vi "main_remote_FPGA.vi"() -> ()   [LabVIEW 2019]
uses:
  <vilib>/platform/TimedLoop/XDataNode/XDataNode.xnode
  <vilib>/Platform/TimedLoop/XDataNode/nitl_modes.ctl
  <vilib>/Platform/TimedLoop/XDataNode/XDNodeRunTimeDep.lvlib
  <vilib>/Platform/TimedLoop/XDataNode/wakeup.ctl
  <vilib>/Platform/TimedLoop/XDataNode/timing_clust.ctl
  FPGA_subVIs/old/motor/motor single class/Variable PID(Kp) mode enum.ctl
  FPGA_subVIs/old/motor/motor single class/Motor single.lvclass
  FPGA_subVIs/old/motor/motor single class/Variable PID(Kp).ctl
  FPGA_subVIs/old/motor/motor enum(FPGA).ctl
panel:
  out "Waveform Chart 2":dbl(graph)
  out "Waveform Chart":cluster{"setpoint":dbl, "encoder out":i32}(graph)
  out "PID out":dbl[](array[numeric])
  out "encoder":i32[](array[numeric])
  out "setpoint":dbl[](array[numeric])
  in  "stop":bool
  out "error out":errorcluster
  in  "error in (no error)":errorcluster
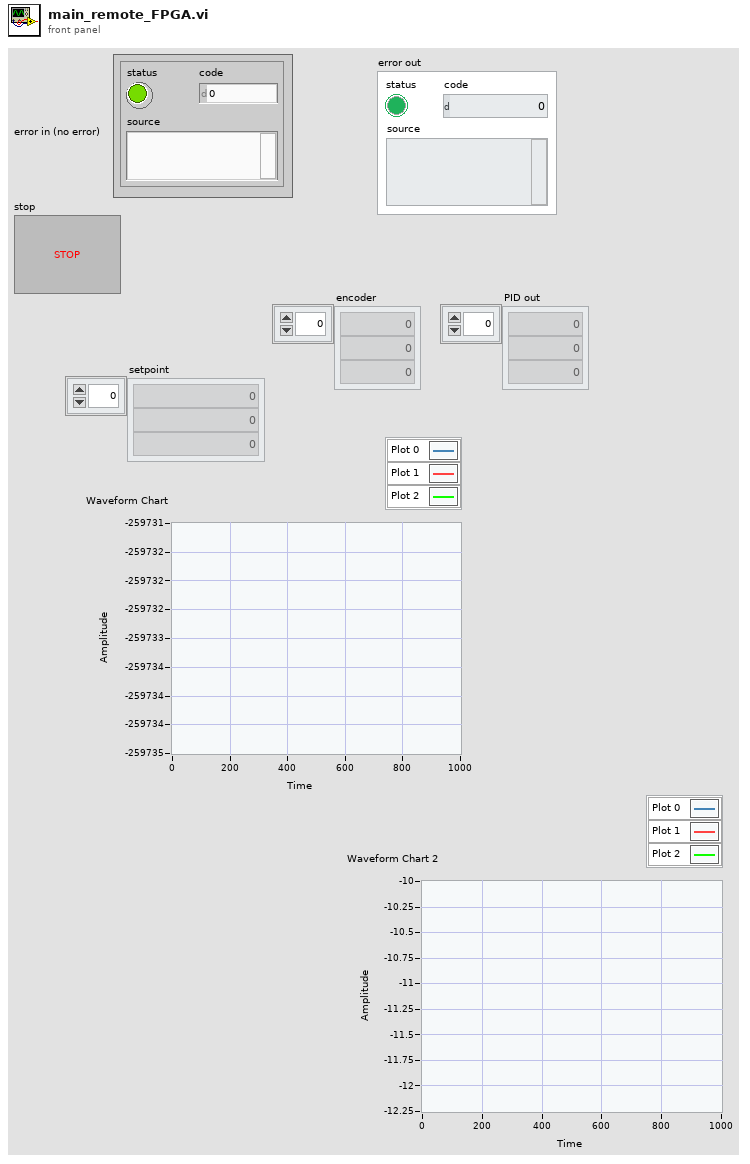
[diagram p1: front panel]
types:
  T1 = typedef "Motor single.lvclass/motor enum(FPGA).ctl" = enum16{"M1", "M2", "M3", "M4"}
  T2 = typedef "Motor single.lvclass/Variable PID(Kp).ctl" = cluster{"Enable variable PID(Kp)":bool, "Variable PID(Kp)range":dbl, "Variable MODE":T3}
  T3 = typedef "Motor single.lvclass/Variable PID(Kp) mode enum.ctl" = enum16{"Log", "Sin&Cos", "Linear", "reverse Log", "const"}
  T4 = typedef "XDNodeRunTimeDep.lvlib/timing_clust.ctl" = cluster{"Expected End [f-1]":u64, "Actual End [f-1]":u64, "Finished Late? [f-1]":bool, "Expected End [i-1]":u64, "Actual End [i-1]":u64, "Finished Late? [i-1]":bool, "Expected Start [i]":u64, "Actual Start [i]":u64, "Expected Start [f]":u64, "Actual Start [f]":u64, "Source Name":string, "Structure Name":string, "Period":i64, "Deadline":i64, "Offset":i64, "Start":i64, "Priority":i32, "Timeout":i32, "Mode":T5, "Wakeup Reason":T6, "Error":errorcluster, "Source Type":string, "Secondary Source Type":string, "Global End Time":u64, "Global Start Time":u64, "Frame Duration":u64, "Iteration Duration":u64, "Assigned CPU":i32, "I/O Scan Engine Mode":u32}
  T5 = typedef "XDNodeRunTimeDep.lvlib/nitl_modes.ctl" = enum32{"No Change", "Process missed periods, maintain original phase", "Discard missed periods, maintain original phase", "Process missed periods, ignore original phase", "Discard missed periods, ignore original phase"}
  T6 = typedef "XDNodeRunTimeDep.lvlib/wakeup.ctl" = enum32{"Normal", "Aborted", "Asynchronous wakeup", "Timing source error", "Timed loop error", "Timeout"}
  T7 = typedef "f710.ctl" = cluster{"Down":bool, "Left":bool, "Up":bool, "Right":bool, "A":bool, "X":bool, "Y":bool, "B":bool, "LB":bool, "RB":bool, "LT":i16, "RT":i16, "L3":bool, "R3":bool, "Ly":i16, "Lx":i16, "Ry":i16, "Rx":i16, "Back":bool, "Start":bool, "center":bool}
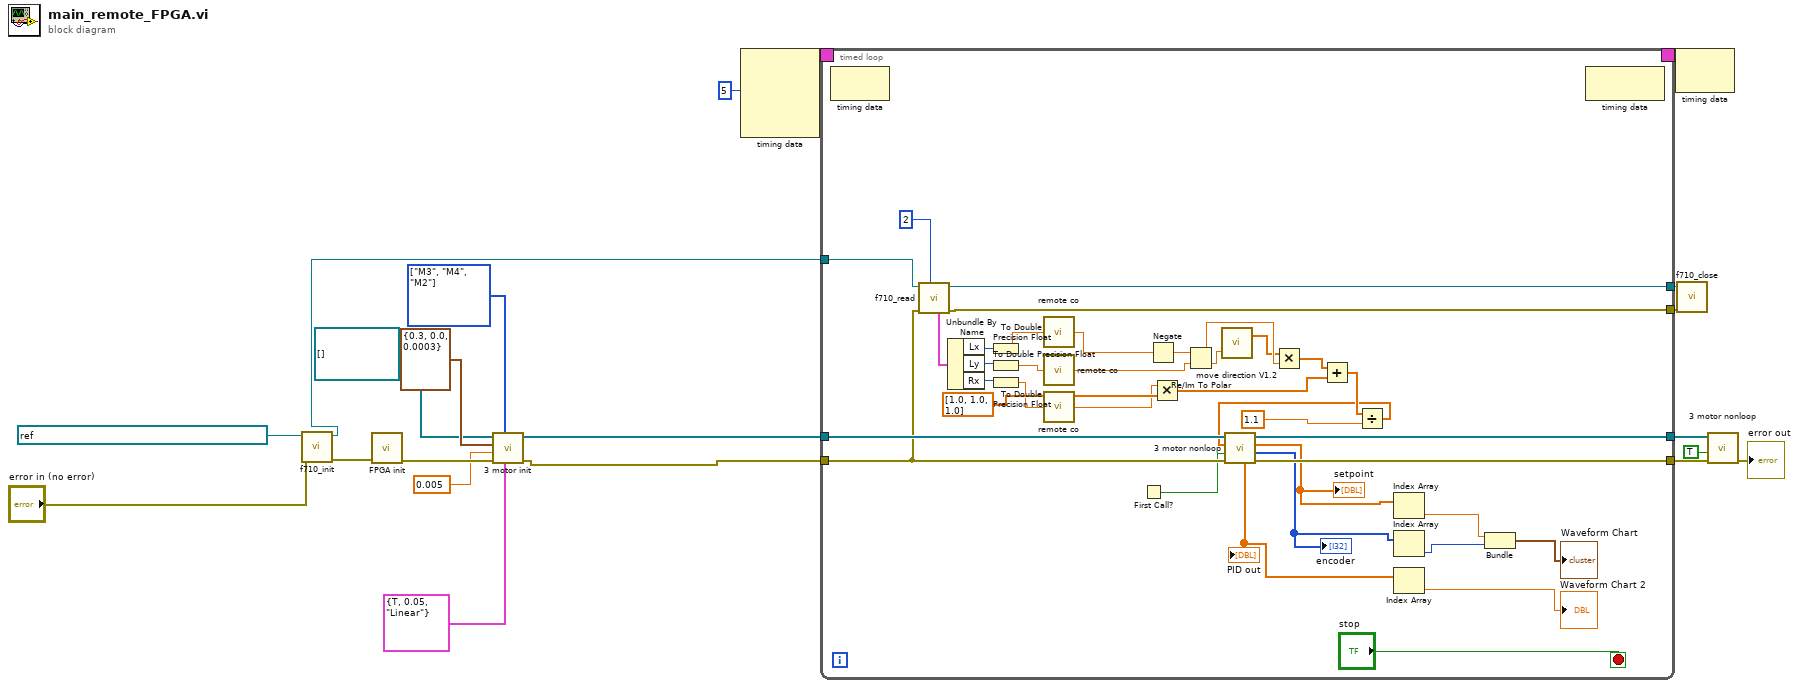
[diagram p0: block diagram]
diagram:
  w12 = T1[] [enum."M3", enum."M4", enum."M2"] items=["M1", "M2", "M3", "M4"] ("Array 2")
  n1 = call <userlib>:"f710_init.vi"("error in (no error)"="error in (no error)", "USB RAW VISA resource name"=refnum<visa-resource-name> "USB0::0x046D::0xC21F::EEAB948F::RAW") -> ("error out"=w5:errorcluster, "VISA Refnum out"=w8:refnum<visa-resource-name>)  [unwired: 8 in]
  n2 = call "FPGA init.vi"("error in"=w5) -> ("error out"=w18:errorcluster)  [unwired: 9 in, 1 out]
  n3 = call "3 motor init.vi"("Variable PID(Kp)"=T2 {"Enable variable PID(Kp)"=TRUE, "Variable PID(Kp)range"=0.05, "Variable MODE"=enum."Linear"}, "Array 2"=w12, "Error In"=w18, "dt(s)"=0.005, "PID"=cluster{"Kp":dbl, "Ki":dbl, "Kd":dbl} {"Kp"=0.3, "Ki"=0.0, "Kd"=0.0003}, "Array"=refnum<class "Motor single.lvclass">[] []) -> ("error out"=w19:errorcluster, "Object array"=w17:refnum<class "Motor single.lvclass">[])  [unwired: 4 in]
  n4 = node-c288(i64 5 ("Period")) -> (w21:T4)  [unwired: 3 in]
  n5 = timed-loop {
    timing: w21 -> [_]
    timing-out: [_] -> w20
    tunnel: w19 -> [w54]
    tunnel: w17 -> [w58]
    tunnel: [w57] -> w11
    tunnel: [w56] -> w10
    tunnel: w8 -> [w55]
    tunnel: [w53] -> w4
    tunnel: [w52] -> w1
    stop <- "stop" stop-if-true
    n6 = node-c288() -> ()  [unwired: 1 in, 1 out]
    n7 = call <userlib>:"f710_read.vi"("Timeout to wait for Interrupt (ms)"=u32 2, "error in (no error)"=w54, "VISA Refnum in"=w55) -> ("error out"=w57:errorcluster, "VISA Refnum out"=w56:refnum<visa-resource-name>, "F710"=w33:T7)  [unwired: 6 in]
    n8 = Unbundle By Name(w33) -> ("Lx"=w51:i16, "Ly"=w50:i16, "Rx"=w49:i16)
    n9 = To Double Precision Float(number=w51) -> (double precision float=w39:dbl)
    n10 = To Double Precision Float(number=w50) -> (double precision float=w37:dbl)
    n11 = To Double Precision Float(number=w49) -> (double precision float=w34:dbl)
    n12 = call "remote co.vi"("input"=w39) -> ("x*y"=w38:dbl)
    n13 = call "remote co.vi"("input"=w37) -> ("x*y"=w36:dbl)
    n14 = call "remote co.vi"("input"=w34) -> ("x*y"=w35:dbl)
    n15 = First Call?() -> (First Call?: T/F=w30:bool)
    n16 = Negate(x=w38) -> (-x=w41:dbl)
    n17 = Multiply(x=w35, y=dbl[] [1.0, 1.0, 1.0]) -> (x*y=w46:dbl[])
    n18 = Re/Im To Polar(2:w36, 3:w41) -> (0:w44:dbl, 1:w43:dbl)
    n19 = call "move direction V1.2.vi"("theta"=w44) -> ("out array"=w42:dbl[])  [unwired: 1 in, 1 out]
    n20 = Multiply(x=w42, y=w43) -> (x*y=w47:dbl[])
    n21 = Add(x=w47, y=w46) -> (x+y=w40:dbl[])
    n22 = Divide(x=w40, y=1.1) -> (x/y=w32:dbl[])
    n23 = call "3 motor nonloop.vi"("Error In"=w54, "Reset"=w30, "speed"=w32, "Array"=w58) -> ("error out"=w53:errorcluster, "encoder"=w27:i32[], "setpoint"=w28:dbl[], "appended array"=w52:refnum<class "Motor single.lvclass">[], "PID out"=w26:dbl[])  [unwired: 3 in]
    "setpoint" <- w28
    "encoder" <- w27
    "PID out" <- w26
    n24 = Index Array(array=w28) -> (element=w25:dbl)  [unwired: 1 in]
    n25 = Index Array(array=w27) -> (element=w24:i32)  [unwired: 1 in]
    n26 = Index Array(array=w26) -> (element=→"Waveform Chart 2":dbl)  [unwired: 1 in]
    n27 = Bundle("setpoint"=w25, "encoder out"=w24) -> (→"Waveform Chart":cluster{"setpoint":dbl, "encoder out":i32})  [unwired: 1 in]
    n28 = node-c288() -> ()  [unwired: 1 in, 1 out]
  }
  n29 = node-c288(w20) -> ()  [unwired: 1 out]
  n30 = call <userlib>:"f710_close.vi"("error in (no error)"=w11, "VISA Refnum in"=w10) -> ()  [unwired: 9 in, 1 out]
  n31 = call "3 motor nonloop.vi"("Error In"=w4, "Reset"=TRUE, "Array"=w1) -> ("error out"=→"error out":errorcluster)  [unwired: 4 in, 4 out]
